vi "LTE_DPD_AMPM_EVM_ACP_UL.vi"() -> ()   [LabVIEW 2016]
doc: "This example illustrates how to use the RFmx SpecAn and LTE personalities together with the RFSG drivers to perform ACP and EVM measurements with or without digital predistortion (DPD) of the waveform input to the DUT. \n\nDPD is a technique to optimize the operating point of power amplifiers and other non-linear RFIC devices. Power amplifiers are much more efficient if they operate near compression. However, compressing signal amplitudes can significantly deteriorate the amplified signal's quality both, in-band (e.g., EVM increases due to non-linear distortion of the signal's I/Q constellation) and out-of-band (e.g., ACP or SEM test fails due to spectral regrowth). With DPD, the original waveform is first pre-distorted in a way that matches the non-linear effects of the RFIC device before being fed through the device. The resulting output is a much cleaner amplified and/or filtered version of the original waveform. \n\nDifferent DPD models can be used to trade off performance with computational ease, with the Lookup-Table (LUT) model the simplest and the Generalized Memory Polynomial Model (GMP) the most complex. With a LUT, the DPD algorithm achieves gain and phase linearization on average. If you want to correct for memory effects - i.e., an output sample not only depends on the current input but also previous input samples; you will notice that a specific input power value translates into a range of gain and phase values - you would use one of the memory polynomial models. For these models, several parameters such as polynomial order and memory depth are available to fine-tune the model to the DUT behavior."
uses:
  Source/SG/Typedefs/Instrument Configuration.ctl
  <instrlib>/niRFSG/niRFSG.llb/niRFSG Ref Clock Sources.ctl
  Source/Common/Local Oscillator Sharing Mode.ctl
  Source/Common/SA Common Configuration.ctl
  <instrlib>/niRFSG/niRFSG.llb/niRFSG Exported Signal Destinations.ctl
  Source/SA/RFmxLTE/Typedefs/LTE Component Carrier Configuration.ctl
  Source/SA/RFmxLTE/Typedefs/LTE ModAcc Configuration.ctl
  Source/SA/RFmxLTE/Typedefs/LTE ACP Configuration.ctl
  Source/SA/RFmxLTE/Typedefs/LTE ACP Offset Results.ctl
  Source/SA/RFmxLTE/Typedefs/LTE ACP Component Carrier Results.ctl
  Source/SA/RFmxSpecAn/Typedefs/SpecAn AMPM Results.ctl
  Source/SA/RFmxSpecAn/Typedefs/SpecAn AMPM Configuration.ctl
  Source/Common/Waveform.ctl
  Source/Methods/RFmxDPD/Typedefs/Common Configuration.ctl
  Source/Methods/RFmxDPD/Typedefs/Memory Polynomial Configuration.ctl
  Source/SA/RFmxInstr/Typedefs/Instrument Configuration.ctl
  Source/Methods/RFmxDPD/Typedefs/Pre DPD Crest Factor Reduction Configuration.ctl
  Source/Methods/RFmxDPD/Typedefs/Pre DPD Crest Factor Reduction Carrier Channel.ctl
  Source/Methods/RFmxDPD/Typedefs/Apply DPD Crest Factor Reduction Configuration.ctl
  Source/Common/SA Auto Level Configuration.ctl
  <vilib>/RFmx/SpecAn/mx/RFmxSpecAn.llb/RFmxSpecAn AMPM Fetch AM to AM Trace.vi
  <vilib>/RFmx/SpecAn/mx/RFmxSpecAn.llb/RFmxSpecAn AMPM Fetch AM to PM Trace.vi
  <vilib>/RFmx/LTE/mx/RFmxLTE.llb/RFmxLTE ModAcc Fetch PUSCH Constellation Trace.vi
  <vilib>/RFmx/LTE/mx/RFmxLTE.llb/RFmxLTE ModAcc Fetch EVM per Subcarrier Trace.vi
  <vilib>/RFmx/LTE/mx/RFmxLTE.llb/RFmxLTE ACP Fetch Absolute Powers Trace.vi
  <vilib>/RFmx/LTE/mx/RFmxLTE.llb/RFmxLTE ACP Fetch Relative Powers Trace.vi
  <vilib>/RFmx/LTE/mx/RFmxLTE.llb/RFmxLTE ACP Fetch Spectrum.vi
  Source/SG/SG.lvlib
  Source/SA/RFmxLTE/RFmxLTE.lvlib
  Source/SA/RFmxSpecAn/RFmxSpecAn.lvlib
  Source/Methods/RFmxDPD/RFmxDPD.lvlib
  Source/SA/RFmxInstr/RFmxInstr.lvlib
  Source/Common/Common.lvlib
panel:
  in  "Error Tab Control":enum32{"Page 1", "Page 2"}(tab)
  out "error out":errorcluster
  in  "Display Tab Control":T1(tab)
  out "AM to PM Plot":T2(graph)
  out "AM to AM Plot":T3(graph)
  out "AMPM Measurement Results":T4 {"AM to PM Residual (deg)" format="%.2f"; "AM to AM Residual (dB)" format="%.2f"; "Mean RMS EVM (%)" format="%.2f"; "1 dB Compression Point (dBm)" format="%.2f"; "Mean Linear Gain (dB)" format="%.2f"}
  out "Constellation Traces":cluster{"DMRS  Constellation":csg[]}[](graph)
  out "EVM Per Subcarrier Trace":cluster{"x0":dbl, "dx":dbl, "y":sgl[]}(graph)
  out "ModAcc Results":T5
  out "ACP Results":T8
  out "Spectrum":cluster{"x0":dbl, "dx":dbl, "y":sgl[]}[](graph)
  out "Reference Waveform":cluster{"t0":dbl, "dt":dbl, "y":sgl[]}(graph)
  in  "Measurement Settings Tab Control":T9(tab)
  in  "RFmx SpecAn AMPM Configuration":T10={"Measurement Interval (s)"=0.0001, "DUT Average Input Power (dBm)"=-20.0, "Signal Type"=0, "Averaging Enabled"=0, "Averaging Count"=10, "Reference Waveform"={"Name"="Wfm", "Data"=refnum, "Signal Bandwidth (Hz)"=0.0, "PAPR (dB)"=0.0, "Burst Length (s)"=0.0, "Sample Rate"=0.0, "Burst Start Locations"=[], "Burst Stop Locations"=[], "Idle Duration Present?"=FALSE, "Runtime Scaling"=0.0, "Script"=""}} {"Reference Waveform"."Runtime Scaling" format="%#_6p"; "Reference Waveform"."Sample Rate" format="%#_6p"; "Reference Waveform"."Burst Length (s)" format="%#_6p"; "Reference Waveform"."PAPR (dB)" format="%.2f"; "Reference Waveform"."Signal Bandwidth (Hz)" format="%#_6p"; "Averaging Enabled" items=["False", "True"]; "Signal Type" items=["Modulated", "Tones"]; "DUT Average Input Power (dBm)" format="%.2f"; "Measurement Interval (s)" format="%.2p"}
  in  "Enable DPD":bool=TRUE
  in  "Common DPD Configuration":T12={"Measurement Interval (s)"=0.0001, "Signal Type"=0, "DUT Average Input Power (dBm)"=-15.0, "Synchronization Method"=1} {"Synchronization Method" items=["Direct"=1, "Alias Protected"=2]; "DUT Average Input Power (dBm)" format="%.2f"; "Signal Type" items=["Modulated", "Tones"]; "Measurement Interval (s)" format="%#.2p"}
  in  "Memory Polynomial Configuration":T13={"Correction Type"=0, "Number of Iterations"=1, " Order"=3, " Depth"=2, "Lead Order"=2, "Lag Order"=2, "Lead Memory Depth"=2, "Lag Memory Depth"=2, "Maximum Lead"=2, "Maximum Lag"=2} {"Order" min=1; "Correction Type" items=["Magnitude and Phase", "Magnitude Only", "Phase Only"]}
  in  "Pre DPD Crest Factor Reduction":T14={"Enabled"=0, "Method"=0, "Max Iterations"=10, "Target PAPR (dB)"=8.0, "Shaping Factor"=5.0, "Shaping Threshold (dB)"=-5.0, "Window Type"=7, "Window Length"=10, "Filter Enabled"=0, "Carrier Channels"=[{"Offset (Hz)"=0.0, "Bandwidth (Hz)"=20000000.0}]} {"Carrier Channels"."Bandwidth (Hz)" format="%.2p"; "Carrier Channels"."Offset (Hz)" format="%.2p"; "Filter Enabled" items=["False", "True"]; "Window Type" items=["Flat Top"=1, "Hanning"=2, "Hamming"=3, "Gaussian"=4, "Blackman"=5, "Blackman-Harris"=6, "Kaiser-Bessel"=7]; "Method" items=["Clipping", "Peak Windowing", "Sigmoid"]; "Enabled" items=["False", "True"]}
  in  "Apply DPD Crest Factor Reduction":T16={"Enabled"=0, "Method"=0, "Max Iterations"=10, "Target PAPR Type"=0, "Target PAPR (dB)"=8.0, "Window Type"=7, "Window Length"=10, "Shaping Factor"=5.0, "Shaping Threshold (dB)"=-5.0} {"Target PAPR Type" items=["Input PAPR", "Custom"]; "Window Type" items=["Flat Top"=1, "Hanning"=2, "Hamming"=3, "Gaussian"=4, "Blackman"=5, "Blackman-Harris"=6, "Kaiser-Bessel"=7]; "Method" items=["Clipping", "Peak Windowing", "Sigmoid"]; "Enabled" items=["False", "True"]}
  in  "ModAcc Configuration":T17={"Synchronization Mode"=1, "Measurement Offset"=0, "Measurement Length"=1, "EVM Unit"=0, "Averaging Enabled"=0, "Averaging Count"=10} {"Averaging Enabled" items=["Percentage", "dB"]; "EVM Unit" items=["Percentage", "dB"]; "Synchronization Mode" items=["Frame", "Slot", "Marker"]}
  in  "ACP Configuration":T18={"Number of GSM Offsets"=0, "Number of UTRA Offsets"=2, "Number of EUTRA Offsets"=1, "Sweep Time Auto"=1, "Sweep Time Interval (s)"=0.001, "Averaging Enabled"=0, "Averaging Count"=10, "Averaging Type"=0, "RBW Auto"=1, "RBW (Hz)"=30000.0, "RBW Filter Type"=0} {"RBW Filter Type" items=["FFT Based", "Gaussian", "Flat"]; "RBW Auto" items=["RMS", "Log", "Scalar", "Max", "Min"]; "Averaging Type" items=["RMS", "Log", "Scalar", "Max", "Min"]; "Averaging Enabled" items=["False", "True"]; "Sweep Time Auto" items=["False", "True"]}
  in  "Center Frequency (Hz)":dbl=1950000000.0 format="%.6p"
  in  "Resource Control":enum32{"RFSG", "RFSA", "LTE Signal"}(tab)
  in  "RFSG Resource Name":refnum<k15>="RFSG"
  in  "Reference Waveform File Path":path=path "C:/Users/Public/Documents/National Instruments/RFIC Test Software/Waveforms/LTE_FDD_UL_1x20MHz_256QAM_OS4.tdms"
  in  "SG Configuration":T19={"SelectedPorts"="", "Reference Clock Source"="PXI_CLK", "Carrier Frequency (Hz)"=1000000000.0, "DUT Average Input Power (dBm)"=-10.0, "External Attenuation (dB)"=0.0, "LO Sharing Mode"=enum."Automatic"}
  in  "Marker Event Output Terminal":T22="PXI_Trig0"
  in  "RFSA Resource Name":refnum<k15>="RFSA"
  in  "Common Configuration":T23={"Center Frequency (Hz)"=1000000000.0, "Reference Level (dBm)"=0.0, "External Attenuation (dB)"=0.0, "Trigger Enabled"=TRUE, "Digital Trigger Source"="PXI_Trig0", "Trigger Delay (s)"=0.0, "Selected Ports"=""} {"Trigger Delay (s)" format="%.2p"; "External Attenuation (dB)" format="%.2f"; "Reference Level (dBm)" format="%.2f"; "Center Frequency (Hz)" format="%.6p"}
  in  "Instrument Configuration":T24={"LO Sharing Mode"=enum."Automatic", "Frequency Reference Source"="PXI_Clk"}
  in  "Auto Level Configuration":T25={"Enabled"=TRUE, "Measurement Interval (s)"=0.01} {"Measurement Interval (s)" min=1e-06 max=100.0 format="%.2p"}
  in  "Signal Configuration":T27={"Link Direction"=1, "Duplex Scheme"=0, "Uplink Downlink Config"=0, "Band"=1, "PUSCH Auto Resource Block Detection Enabled"=1, "Auto DMRS Detection Enabled"=0, "Downlink Auto Cell ID Detection Enabled"=0, "Component Carrier Configurations"=[{"Bandwidth (Hz)"=20000000.0, "Cell ID"=0, "PUSCH Modulation Type"=3, "PUSCH Resource Block Offset"=0, "PUSCH Number of Resource Blocks"=-1, "Downlink Test Model"=0}]} {"Downlink Auto Cell ID Detection Enabled" items=["False", "True"]; "Link Direction" items=["Downlink", "Uplink"]; "Auto DMRS Detection Enabled" items=["False", "True"]; "PUSCH Auto Resource Block Detection Enabled" items=["False", "True"]; "Component Carrier Configurations"."Downlink Test Model" items=["TM1.1", "TM1.2", "TM2", "TM 2a", "TM 3.1", "TM 3.2", "TM 3.3", "TM 3.1a"]; "Component Carrier Configurations"."PUSCH Modulation Type" items=["QPSK", "16 QAM", "64 QAM", "256 QAM", "1024 QAM"]; "Component Carrier Configurations"."Bandwidth (Hz)" items=["200.0 k"=200000.0, "1.4 M"=1400000.0, "3.0 M"=3000000.0, "5.0 M"=5000000.0, "10.0 M"=10000000.0, "15.0 M"=15000000.0, "20.0 M"=20000000.0]; "Uplink Downlink Config" items=["0", "1", "2", "3", "4", "5", "6"]; "Duplex Scheme" items=["FDD", "TDD", "LAA"]}
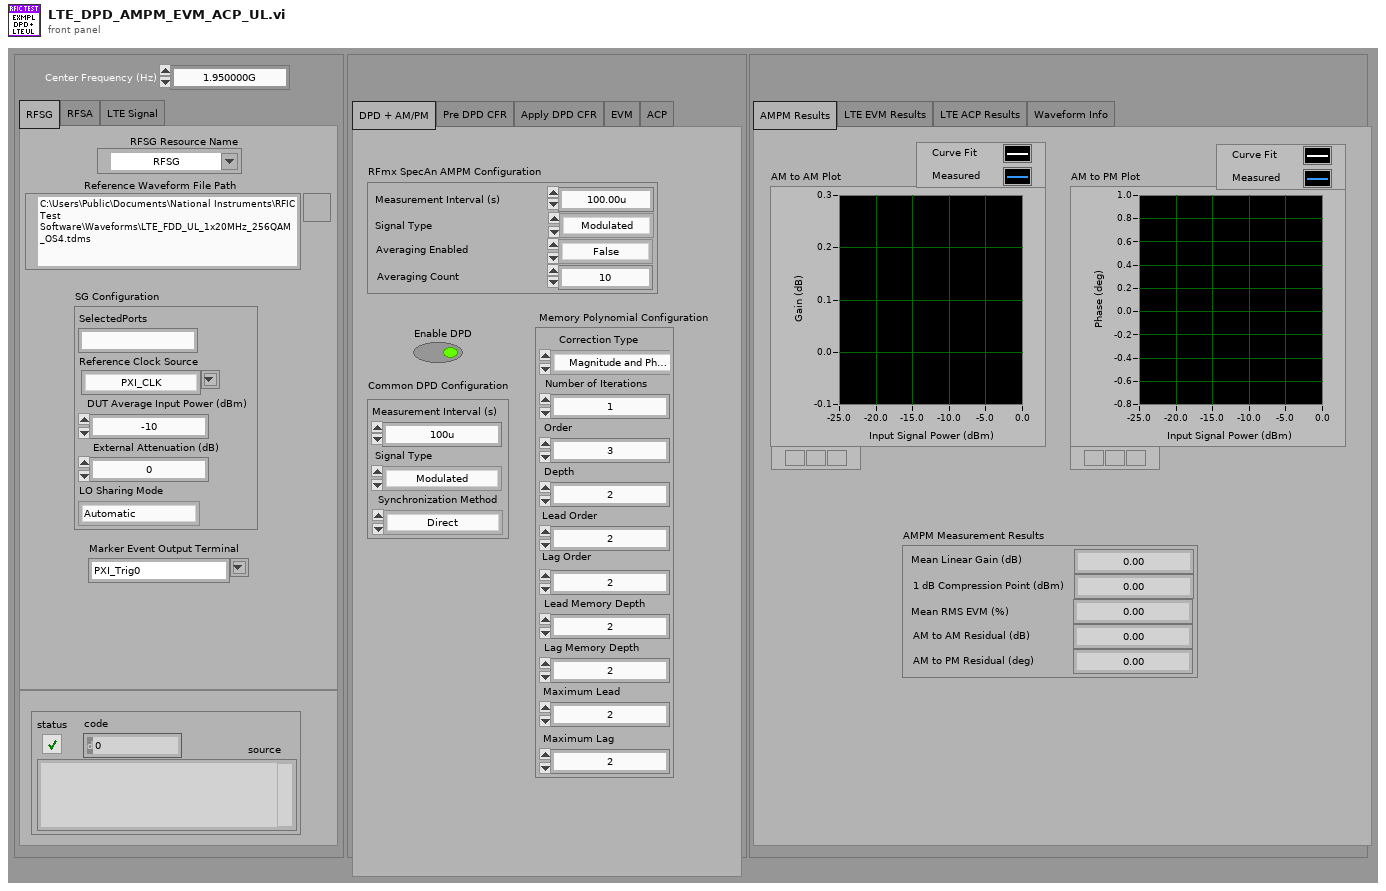
[diagram p1: front panel]
types:
  T1 = enum32{"AMPM Results", "LTE EVM Results", "LTE ACP Results", "Waveform Info"}
  T2 = cluster{"Input Powers (dBm)":sgl[], "Curve Fit AM to PM (dB)":sgl[]}[]
  T3 = cluster{"Input Powers (dBm)":sgl[], "Curve Fit AM to AM (dB)":sgl[]}[]
  T4 = typedef "RFmxSpecAn.lvlib/SpecAn AMPM Results.ctl" = cluster{"Mean Linear Gain (dB)":dbl, "1 dB Compression Point (dBm)":dbl, "Mean RMS EVM (%)":dbl, "AM to AM Residual (dB)":dbl, "AM to PM Residual (deg)":dbl}
  T5 = cluster{"Component Carrier Results":cluster{"Peak Composite EVM Subcarrier Index":i32, "Peak Composite EVM Symbol Index":i32, "Mean RMS Composite EVM":dbl, "Max Peak Composite EVM":dbl, "Mean Frequency Error (Hz)":dbl, "Peak Composite EVM Slot Index":i32}[]}
  T6 = typedef "RFmxLTE.lvlib/LTE ACP Offset Results.ctl" = cluster{"Lower Absolute Power (dBm)":dbl, "Upper Absolute Power (dBm)":dbl, "Lower Relative Power (dB)":dbl, "Upper Relative Power (dB)":dbl, "Frequency (Hz)":dbl, "Integration Bandwidth (Hz)":dbl}
  T7 = typedef "RFmxLTE.lvlib/LTE ACP Component Carrier Results.ctl" = cluster{"Absolute Power (dBm)":dbl, "Relative Power (dB)":dbl}
  T8 = cluster{"Offset Results":T6[], "Component Carrier Results":T7[]}
  T9 = enum32{"DPD + AM/PM", "Pre DPD CFR", "Apply DPD CFR", "EVM", "ACP"}
  T10 = typedef "RFmxSpecAn.lvlib/SpecAn AMPM Configuration.ctl" = cluster{"Measurement Interval (s)":dbl, "DUT Average Input Power (dBm)":dbl, "Signal Type":i32, "Averaging Enabled":i32, "Averaging Count":i32, "Reference Waveform":T11}
  T11 = typedef "Common.lvlib/Waveform.ctl" = cluster{"Name":string, "Data":refnum<data-value>, "Signal Bandwidth (Hz)":dbl, "PAPR (dB)":dbl, "Burst Length (s)":dbl, "Sample Rate":dbl, "Burst Start Locations":i32[], "Burst Stop Locations":i32[], "Idle Duration Present?":bool, "Runtime Scaling":dbl, "Script":string}
  T12 = typedef "RFmxDPD.lvlib/Common Configuration.ctl" = cluster{"Measurement Interval (s)":dbl, "Signal Type":i32, "DUT Average Input Power (dBm)":dbl, "Synchronization Method":i32}
  T13 = typedef "RFmxDPD.lvlib/Memory Polynomial Configuration.ctl" = cluster{"Correction Type":i32, "Number of Iterations":i32, " Order":i32, " Depth":i32, "Lead Order":i32, "Lag Order":i32, "Lead Memory Depth":i32, "Lag Memory Depth":i32, "Maximum Lead":i32, "Maximum Lag":i32}
  T14 = typedef "RFmxDPD.lvlib/Pre DPD Crest Factor Reduction Configuration.ctl" = cluster{"Enabled":i32, "Method":i32, "Max Iterations":i32, "Target PAPR (dB)":dbl, "Shaping Factor":dbl, "Shaping Threshold (dB)":dbl, "Window Type":i32, "Window Length":i32, "Filter Enabled":i32, "Carrier Channels":T15[]}
  T15 = typedef "RFmxDPD.lvlib/Pre DPD Crest Factor Reduction Carrier Channel.ctl" = cluster{"Offset (Hz)":dbl, "Bandwidth (Hz)":dbl}
  T16 = typedef "RFmxDPD.lvlib/Apply DPD Crest Factor Reduction Configuration.ctl" = cluster{"Enabled":i32, "Method":i32, "Max Iterations":i32, "Target PAPR Type":i32, "Target PAPR (dB)":dbl, "Window Type":i32, "Window Length":i32, "Shaping Factor":dbl, "Shaping Threshold (dB)":dbl}
  T17 = typedef "RFmxLTE.lvlib/LTE ModAcc Configuration.ctl" = cluster{"Synchronization Mode":i32, "Measurement Offset":i32, "Measurement Length":i32, "EVM Unit":i32, "Averaging Enabled":i32, "Averaging Count":i32}
  T18 = typedef "RFmxLTE.lvlib/LTE ACP Configuration.ctl" = cluster{"Number of GSM Offsets":i32, "Number of UTRA Offsets":i32, "Number of EUTRA Offsets":i32, "Sweep Time Auto":i32, "Sweep Time Interval (s)":dbl, "Averaging Enabled":i32, "Averaging Count":i32, "Averaging Type":i32, "RBW Auto":i32, "RBW (Hz)":dbl, "RBW Filter Type":i32}
  T19 = typedef "SG.lvlib/Instrument Configuration.ctl" = cluster{"SelectedPorts":string, "Reference Clock Source":T20, "Carrier Frequency (Hz)":dbl, "DUT Average Input Power (dBm)":dbl, "External Attenuation (dB)":dbl, "LO Sharing Mode":T21}
  T20 = typedef "niRFSG Ref Clock Sources.ctl" = string
  T21 = typedef "Common.lvlib/Local Oscillator Sharing Mode.ctl" = enum16{"Automatic", "None"}
  T22 = typedef "niRFSG Exported Signal Destinations.ctl" = string
  T23 = typedef "Common.lvlib/SA Common Configuration.ctl" = cluster{"Center Frequency (Hz)":dbl, "Reference Level (dBm)":dbl, "External Attenuation (dB)":dbl, "Trigger Enabled":bool, "Digital Trigger Source":string, "Trigger Delay (s)":dbl, "Selected Ports":string}
  T24 = typedef "RFmxInstr.lvlib/Instrument Configuration.ctl" = cluster{"LO Sharing Mode":T21, "Frequency Reference Source":string}
  T25 = typedef "Common.lvlib/SA Auto Level Configuration.ctl" = cluster{"Enabled":bool, "Measurement Interval (s)":dbl}
  T26 = typedef "RFmxLTE.lvlib/LTE Component Carrier Configuration.ctl" = cluster{"Bandwidth (Hz)":dbl, "Cell ID":i32, "PUSCH Modulation Type":i32, "PUSCH Resource Block Offset":i32, "PUSCH Number of Resource Blocks":i32, "Downlink Test Model":i32}
  T27 = cluster{"Link Direction":i32, "Duplex Scheme":i32, "Uplink Downlink Config":i32, "Band":i32, "PUSCH Auto Resource Block Detection Enabled":i32, "Auto DMRS Detection Enabled":i32, "Downlink Auto Cell ID Detection Enabled":i32, "Component Carrier Configurations":T26[]}
  T28 = enum16{"ACP", "CHP", "ModAcc", "OBW", "SEM", "PVT", "SlotPhase", "SlotPower"}[]
  T29 = enum16{"ACP", "CCDF", "CHP", "FCnt", "Harmonics", "OBW", "SEM", "Spectrum", "Spur", "TXP", "AMPM", "DPD", "IQ", "IM", "NF", "PhaseNoise", "PAVT"}[]
  T30 = cluster{"Reference Powers (dBm)":sgl[], "Measured AM to PM (deg)":sgl[]}
  T31 = cluster{"Reference Powers (dBm)":sgl[], "Curve Fit AM to AM (dB)":sgl[]}
  T32 = cluster{"Reference Powers (dBm)":sgl[], "Measured AM to AM (dB)":sgl[]}
  T33 = cluster{"Reference Powers (dBm)":sgl[], "Curve Fit AM to PM (deg)":sgl[]}
  T34 = cluster{"Reference Powers (dBm)":sgl[], "Measured AM to AM (dB)":sgl[]}[]
  T35 = cluster{"Reference Powers (dBm)":sgl[], "Measured AM to PM (deg)":sgl[]}[]
  T36 = typedef "RFmxLTE.lvlib/LTE ModAcc Results.ctl" = cluster{"Component Carrier Results":T37[]}
  T37 = typedef "RFmxLTE.lvlib/LTE ModAcc Component Carrier Results.ctl" = cluster{"Peak Composite EVM Subcarrier Index":i32, "Peak Composite EVM Symbol Index":i32, "Mean RMS Composite EVM":dbl, "Max Peak Composite EVM":dbl, "Mean Frequency Error (Hz)":dbl, "Peak Composite EVM Slot Index":i32}
  T38 = typedef "RFmxLTE.lvlib/LTE ACP Results.ctl" = cluster{"Offset Results":T6[], "Component Carrier Results":T7[]}
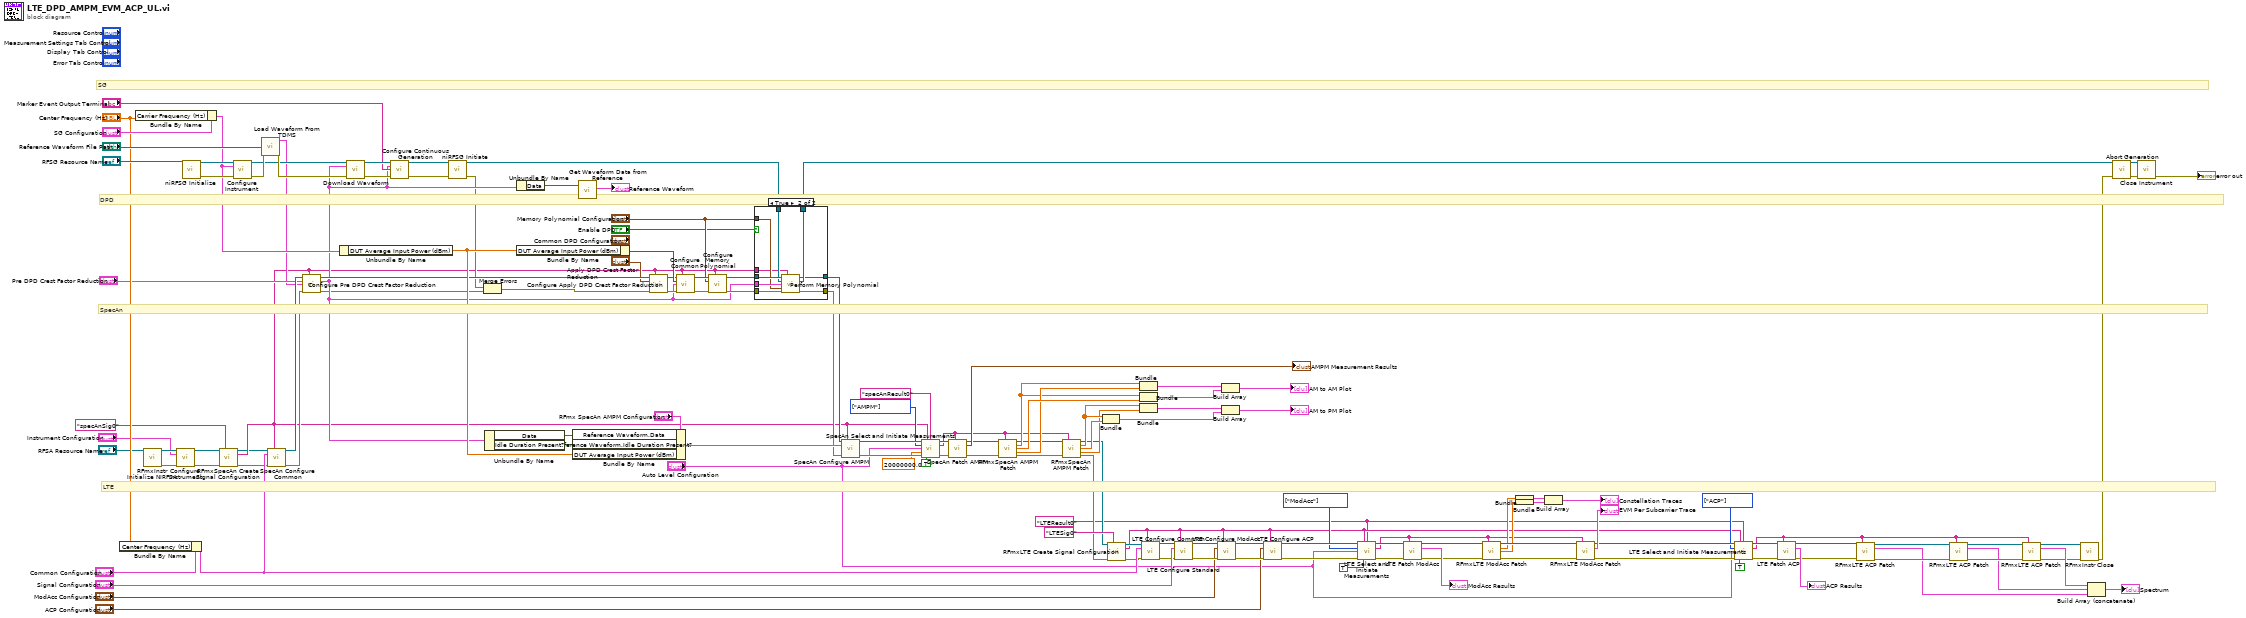
[diagram p0: block diagram]
diagram:
  w5 = "LTEResult0"
  w24 = T28 [enum."ACP"] items=["ACP", "CHP", "ModAcc", "OBW", "SEM", "PVT", "SlotPhase", "SlotPower"] ("Measurements")
  w29 = T28 [enum."ModAcc"] items=["ACP", "CHP", "ModAcc", "OBW", "SEM", "PVT", "SlotPhase", "SlotPower"] ("Measurements")
  w36 = T29 [enum."AMPM"] items=["ACP", "CCDF", "CHP", "FCnt", "Harmonics", "OBW", "SEM", "Spectrum", "Spur", "TXP", "AMPM", "DPD", "IQ", "IM", "NF", "PhaseNoise", "PAVT"] ("Measurements")
  # "SpecAn"
  # "LTE"
  # "DPD"
  # "SG"
  n1 = Bundle By Name(cluster="Common Configuration", "Center Frequency (Hz)"="Center Frequency (Hz)") -> (w58:T23)
  n2 = Bundle By Name(cluster="SG Configuration", "Carrier Frequency (Hz)"="Center Frequency (Hz)") -> (w129:T19)
  n3 = call <vilib>:"RFmxInstr Initialize NIRFSA.vi"("Resource Name"="RFSA Resource Name") -> ("Instrument Handle Out"=w57:refnum<k21>, "error out"=w56:errorcluster)  [unwired: 12 in, 1 out]
  n4 = call "Configure Instrument.vi"("Instrument Handle In"=w57, "Instrument Configuration"="Instrument Configuration", "error in (no error)"=w56) -> ("Instrument Handle Out"=w4:refnum<k21>, "error out"=w1:errorcluster)  [unwired: 11 in]
  n5 = call <instrlib>:"niRFSG Initialize.vi"("resource name"="RFSG Resource Name") -> ("instrument handle"=w140:refnum<k15>, "error out"=w139:errorcluster)  [unwired: 13 in]
  n6 = call <vilib>:"RFmxSpecAn Create Signal Configuration.vi"("Instrument Handle In"=w4, "Signal Name"="specAnSig0", "error in (no error)"=w1) -> ("Instrument Handle Out"=w3:refnum<k21>, "Selector String Out"=w16:string, "error out"=w2:errorcluster)  [unwired: 10 in]
  n7 = call "Configure Instrument.vi"("RFSG Session In"=w140, "SG Configuration"=w129, "error in (no error)"=w139) -> ("RFSG Session Out"=w141:refnum<k15>, "error out"=w143:errorcluster)  [unwired: 11 in]
  n8 = call "Load Waveform From TDMS.vi"("TDMS File Path"="Reference Waveform File Path", "error in (no error)"=w143) -> ("Waveform"=w44:T11, "error out"=w142:errorcluster)  [unwired: 12 in]
  n9 = call "SpecAn Configure Common.vi"("RFmx Handle In"=w3, "Selector String"=w16, "Common Configuration"=w58, "error in (no error)"=w2) -> ("RFmx Handle Out"=w49:refnum<k21>, "error out"=w50:errorcluster)  [unwired: 10 in]
  n10 = call "Configure Pre DPD Crest Factor Reduction.vi"("Instrument Handle In"=w49, "Selector String"=w16, "Pre DPD Crest Factor Reduction Configuration"="Pre DPD Crest Factor Reduction", "Reference Waveform"=w44, "error in (no error)"=w50) -> ("Instrument Handle Out"=w51:refnum<k21>, "Pre DPD CFR Waveform"=w21:T11, "error out"=w20:errorcluster)  [unwired: 8 in]
  n11 = Unbundle By Name(w129) -> ("DUT Average Input Power (dBm)"=w63:dbl)
  n12 = call "Download Waveform.vi"("RFSG handle"=w141, "Waveform In"=w21, "error in (no error)"=w142) -> ("RFSG handle out"=w136:refnum<k15>, "error out"=w135:errorcluster)  [unwired: 11 in]
  n13 = call "Configure Continuous Generation.vi"("RFSG handle"=w136, "Waveform in"=w21, "Waveform Start Trigger Export"="Marker Event Output Terminal", "error in"=w135) -> ("RFSG handle out"=w137:refnum<k15>, "error out"=w138:errorcluster)  [unwired: 9 in, 1 out]
  n14 = call <instrlib>:"niRFSG Initiate.vi"("instrument handle"=w137, "error in"=w138) -> ("instrument handle out"=w67:refnum<k15>, "error out"=w18:errorcluster)  [unwired: 12 in]
  n15 = Merge Errors(w18, w20) -> (w19:errorcluster)
  n16 = Unbundle By Name(w21) -> ("Data"=w131:refnum<data-value>, "Idle Duration Present?"=w130:bool)
  n17 = Unbundle By Name(w21) -> ("Data"=w43:refnum<data-value>)
  n18 = Bundle By Name(cluster="Common DPD Configuration", "DUT Average Input Power (dBm)"=w63) -> (w64:T12)
  n19 = Bundle By Name(cluster="RFmx SpecAn AMPM Configuration", "Reference Waveform.Data"=w131, "Reference Waveform.Idle Duration Present?"=w130, "DUT Average Input Power (dBm)"=w63) -> (w91:T10)
  n20 = call "Get Waveform Data from Reference.vi"("Waveform Data Reference"=w43) -> ("Waveform Data"=→"Reference Waveform":cluster{"t0":dbl, "dt":dbl, "y":csg[]})  [unwired: 13 in, 1 out]
  n21 = call "Configure Apply DPD Crest Factor Reduction.vi"("Instrument Handle In"=w51, "Selector String"=w16, "Apply DPD Crest Factor Reduction Configuration"="Apply DPD Crest Factor Reduction", "error in (no error)"=w19) -> ("Instrument Handle Out"=w45:refnum<k21>, "error out"=w46:errorcluster)  [unwired: 10 in]
  n22 = call "Configure Common.vi"("Instrument Handle In"=w45, "Selector String"=w16, "Common Configuration"=w64, "Reference Waveform"=w21, "error in (no error)"=w46) -> ("Instrument Handle Out"=w73:refnum<k21>, "error out"=w72:errorcluster)  [unwired: 9 in]
  n23 = call "Configure Memory Polynomial.vi"("Instrument Handle In"=w73, "Selector String"=w16, "Memory Polynomial Configuration"="Memory Polynomial Configuration", "error in (no error)"=w72) -> ("Instrument Handle Out"=w71:refnum<k21>, "error out"=w70:errorcluster)  [unwired: 10 in]
  n24 = case shown="True" "Enable DPD" {
    tunnel: w71 -> [w145 w155]
    tunnel: [w144 w154] -> w60
    tunnel: "Memory Polynomial Configuration" -> [_ w148]
    tunnel: w21 -> [_ w153]
    tunnel: w67 -> [w146 w152]
    tunnel: [w146 w151] -> w66
    tunnel: [w145 w150] -> w59
    tunnel: w70 -> [w144 w149]
    tunnel: w16 -> [_ w147]
    frame False {
    }
    frame True {
      n25 = call "Perform Memory Polynomial.vi"("RFmx Instrument Handle In"=w155, "Selector String"=w147, "RFSG Instrument Handle In"=w152, "Reference Waveform"=w153, "Memory Polynomial Configuration"=w148, "error in (no error)"=w149) -> ("RFmx Instrument Handle Out"=w150:refnum<k21>, "RFSG Instrument Handle Out"=w151:refnum<k15>, "error out"=w154:errorcluster)  [unwired: 6 in, 1 out]
    }
  }
  n26 = call "SpecAn Configure AMPM.vi"("RFmx Handle In"=w59, "Selector String"=w16, "RFmx SpecAn AMPM Configuration"=w91, "error in (no error)"=w60) -> ("RFmx Handle Out"=w41:refnum<k21>, "error out"=w39:errorcluster)  [unwired: 10 in]
  n27 = call "SpecAn Select and Initiate Measurements.vi"("Instrument Handle In"=w41, "Selector String"=w16, "Result Name"="specAnResult0", "Measurements"=w36, "Auto Level Configuration"="Auto Level Configuration", "Auto Level Bandwidth (Hz)"=20000000.0, "error in (no error)"=w39, "Enable All Traces (F)"=TRUE) -> ("Instrument Handle Out"=w40:refnum<k21>, "Selector String Out"=w15:string, "error out"=w38:errorcluster)  [unwired: 5 in]
  n28 = call "SpecAn Fetch AMPM.vi"("RFmx Handle In"=w40, "Selector String"=w15, "error in (no error)"=w38) -> ("RFmx Handle Out"=w77:refnum<k21>, "AMPM Results"=→"AMPM Measurement Results":T4, "error out"=w76:errorcluster)  [unwired: 10 in]
  n29 = call-poly <vilib>:"RFmxSpecAn AMPM Fetch.vi"("Instrument Handle In"=w77, "Selector String"=w15, "error in (no error)"=w76) -> ("Instrument Handle Out"=w83:refnum<k21>, "Reference Powers (dBm)"=w87:sgl[], "Measured AM to AM (dB)"=w89:sgl[], "Curve Fit AM to AM (dB)"=w88:sgl[], "error out"=w82:errorcluster)  [unwired: 8 in]
  n30 = call-poly <vilib>:"RFmxSpecAn AMPM Fetch.vi"("Instrument Handle In"=w83, "Selector String"=w15, "error in (no error)"=w82) -> ("Instrument Handle Out"=w11:refnum<k21>, "Reference Powers (dBm)"=w86:sgl[], "Measured AM to PM (deg)"=w85:sgl[], "Curve Fit AM to PM (deg)"=w84:sgl[], "error out"=w12:errorcluster)  [unwired: 8 in]
  n31 = Bundle("Reference Powers (dBm)"=w86, "Measured AM to PM (deg)"=w85) -> (w79:T30)  [unwired: 1 in]
  n32 = call <vilib>:"RFmxLTE Create Signal Configuration.vi"("Instrument Handle In"=w11, "Signal Name"="LTESig0", "error in (no error)"=w12) -> ("Instrument Handle Out"=w10:refnum<k21>, "Selector String Out"=w7:string, "error out"=w9:errorcluster)  [unwired: 10 in]
  n33 = Bundle("Reference Powers (dBm)"=w87, "Curve Fit AM to AM (dB)"=w88) -> (w81:T31)  [unwired: 1 in]
  n34 = Bundle("Reference Powers (dBm)"=w87, "Measured AM to AM (dB)"=w89) -> (w80:T32)  [unwired: 1 in]
  n35 = Bundle("Reference Powers (dBm)"=w86, "Curve Fit AM to PM (deg)"=w84) -> (w78:T33)  [unwired: 1 in]
  n36 = call "LTE Configure Common.vi"("RFmx Handle In"=w10, "Selector String"=w7, "Common Configuration"=w58, "error in (no error)"=w9) -> ("RFmx Handle Out"=w69:refnum<k21>, "error out"=w68:errorcluster)  [unwired: 10 in]
  n37 = call "LTE Configure Standard.vi"("RFmx Handle In"=w69, "Selector String"=w7, "LTE Standard Configuration"="Signal Configuration", "error in (no error)"=w68) -> ("RFmx Handle Out"=w119:refnum<k21>, "error out"=w120:errorcluster)  [unwired: 10 in]
  n38 = call "LTE Configure ModAcc.vi"("RFmx Handle In"=w119, "Selector String"=w7, "ModAcc Configuration"="ModAcc Configuration", "error in (no error)"=w120) -> ("RFmx Handle Out"=w118:refnum<k21>, "error out"=w117:errorcluster)  [unwired: 10 in]
  n39 = Build Array(w81, w80) -> (→"AM to AM Plot":T34)
  n40 = Build Array(w78, w79) -> (→"AM to PM Plot":T35)
  n41 = call "LTE Configure ACP.vi"("RFmx Handle In"=w118, "Selector String"=w7, "ACP Configuration"="ACP Configuration", "error in (no error)"=w117) -> ("RFmx Handle Out"=w34:refnum<k21>, "error out"=w33:errorcluster)  [unwired: 10 in]
  n42 = call "LTE Select and Initiate Measurements.vi"("Instrument Handle In"=w34, "Selector String"=w7, "Result Name"=w5, "Measurements"=w29, "Auto Level Configuration"="Auto Level Configuration", "error in (no error)"=w33, "Enable All Traces (F)"=TRUE) -> ("Instrument Handle Out"=w31:refnum<k21>, "Selector String Out"=w8:string, "error out"=w32:errorcluster)  [unwired: 6 in]
  n43 = call "LTE Fetch ModAcc.vi"("RFmx Handle In"=w31, "Selector String"=w8, "error in (no error)"=w32) -> ("RFmx Handle Out"=w105:refnum<k21>, "ModAcc Results"=→"ModAcc Results":T36, "error out"=w104:errorcluster)  [unwired: 10 in]
  n44 = call-poly <vilib>:"RFmxLTE ModAcc Fetch.vi"("Instrument Handle In"=w105, "Selector String"=w8, "error in (no error)"=w104) -> ("Instrument Handle Out"=w113:refnum<k21>, "Data Constellation"=w110:csg[], "DMRS  Constellation"=w109:csg[], "error out"=w112:errorcluster)  [unwired: 9 in]
  n45 = Bundle("Data Constellation"=w110) -> (w108:cluster{"Data Constellation":csg[]})  [unwired: 1 in]
  n46 = Bundle("DMRS  Constellation"=w109) -> (w107:cluster{"DMRS  Constellation":csg[]})  [unwired: 1 in]
  n47 = Build Array(w108, w107) -> (→"Constellation Traces":cluster{"DMRS  Constellation":csg[]}[])
  n48 = call-poly <vilib>:"RFmxLTE ModAcc Fetch.vi"("Instrument Handle In"=w113, "Selector String"=w8, "error in (no error)"=w112) -> ("Instrument Handle Out"=w28:refnum<k21>, "Mean RMS EVM per Subcarrier (% or dB)"=→"EVM Per Subcarrier Trace":cluster{"x0":dbl, "dx":dbl, "y":sgl[]}, "error out"=w25:errorcluster)  [unwired: 10 in]
  n49 = call "LTE Select and Initiate Measurements.vi"("Instrument Handle In"=w28, "Selector String"=w7, "Result Name"=w5, "Measurements"=w24, "Auto Level Configuration"="Auto Level Configuration", "error in (no error)"=w25, "Enable All Traces (F)"=TRUE) -> ("Instrument Handle Out"=w27:refnum<k21>, "Selector String Out"=w6:string, "error out"=w26:errorcluster)  [unwired: 6 in]
  n50 = call "LTE Fetch ACP.vi"("RFmx Handle In"=w27, "Selector String"=w6, "error in (no error)"=w26) -> ("RFmx Handle Out"=w95:refnum<k21>, "ACP Results"=→"ACP Results":T38, "error out"=w94:errorcluster)  [unwired: 10 in]
  n51 = call-poly <vilib>:"RFmxLTE ACP Fetch.vi"("Instrument Handle In"=w95, "Selector String"=w6, "error in (no error)"=w94) -> ("Instrument Handle Out"=w103:refnum<k21>, "Absolute Powers (dBm)"=w97:cluster{"x0":dbl, "dx":dbl, "y":sgl[]}[], "error out"=w101:errorcluster)  [unwired: 10 in]
  n52 = call-poly <vilib>:"RFmxLTE ACP Fetch.vi"("Instrument Handle In"=w103, "Selector String"=w6, "error in (no error)"=w101) -> ("Instrument Handle Out"=w102:refnum<k21>, "Relative Powers (dB)"=w98:cluster{"x0":dbl, "dx":dbl, "y":sgl[]}[], "error out"=w100:errorcluster)  [unwired: 10 in]
  n53 = call-poly <vilib>:"RFmxLTE ACP Fetch.vi"("Instrument Handle In"=w102, "Selector String"=w6, "error in (no error)"=w100) -> ("Instrument Handle Out"=w53:refnum<k21>, "Spectrum (dBm)"=w99:cluster{"x0":dbl, "dx":dbl, "y":sgl[]}, "error out"=w54:errorcluster)  [unwired: 10 in]
  n54 = call <vilib>:"RFmxInstr Close.vi"("Instrument Handle In"=w53, "error in (no error)"=w54) -> ("error out"=w52:errorcluster)  [unwired: 13 in]
  n55 = Build Array (concatenate)(w99, w98, w97) -> (→"Spectrum":cluster{"x0":dbl, "dx":dbl, "y":sgl[]}[])
  n56 = call "Abort Generation.vi"("RFSG handle"=w66, "error in (no error)"=w52) -> ("RFSG handle out"=w123:refnum<k15>, "error out"=w124:errorcluster)  [unwired: 12 in]
  n57 = call "Close Instrument.vi"("RFSG Handle"=w123, "error in (no error)"=w124) -> ("error out"=→"error out":errorcluster)  [unwired: 13 in]
